vi "索引数据.vi"(5 "数据":T2[](array[typedef]), 6 "显示曲线范围":T3, 7 "显示数据":i32[](array[numeric]), 8 "测试类型":T1 caption="数据", 11 "索引簇":T4 {"索引" min=0}) -> (3 "数组":T5[](array[typedef]), 4 "当前索引":T2)   [LabVIEW 2020]
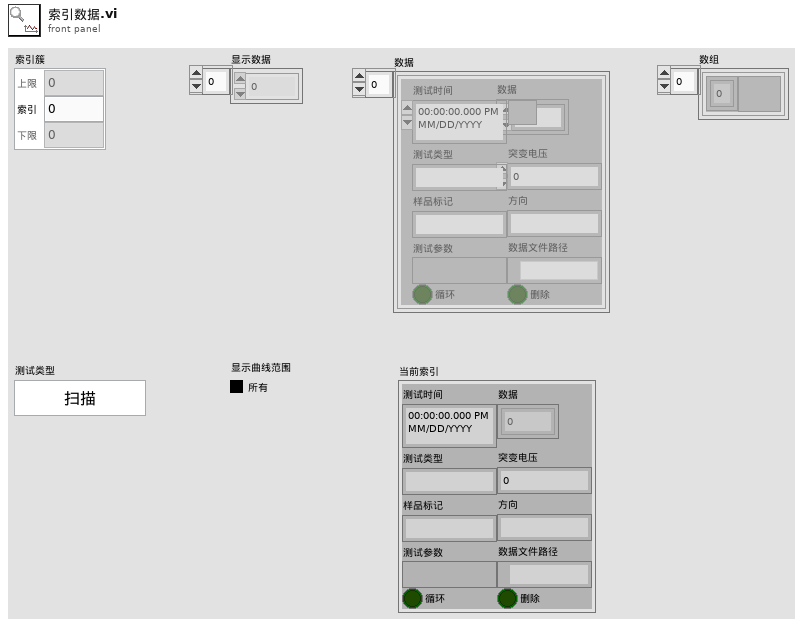
[diagram p1: front panel]
types:
  T1 = typedef "测试类型.ctl" = enum16{"扫描", "保持时间", "脉冲", "高速脉冲", "任意波形"}
  T2 = typedef "测试数据类型.ctl" = cluster{"测试时间":timestamp, "测试类型":string, "样品标记":string, "测试参数":variant, "循环":bool, "数据":dbl[][], "删除":bool, "突变电压":i32, "方向":string, "数据文件路径":path}
  T3 = typedef "显示曲线范围.ctl" = enum8{"False", "True", "Mixed"}
  T4 = typedef "索引簇.ctl" = cluster{"上限":i32, "索引":i32, "下限":i32}
  T5 = typedef "数据显示.xctl/波形数据定义.ctl" = cluster{"波形":dbl[][], "属性":variant}
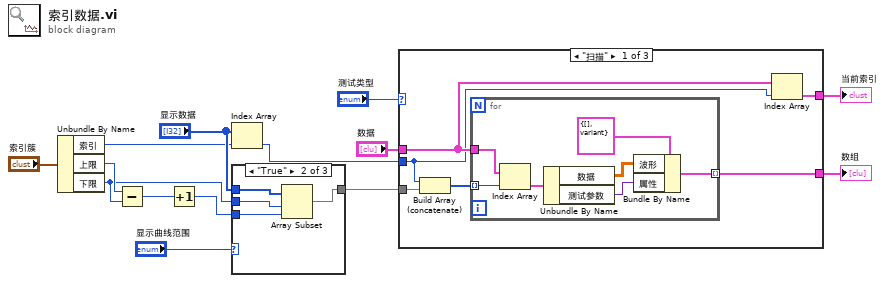
[diagram p0: block diagram]
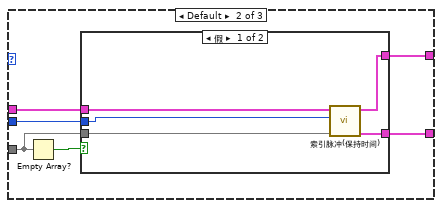
[diagram p2: hidden frame]
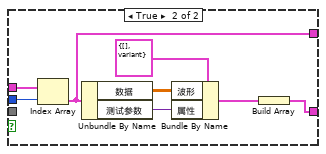
[diagram p3: hidden frame]
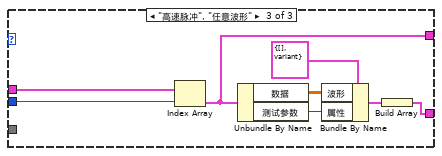
[diagram p4: hidden frame]
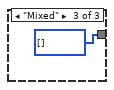
[diagram p6: hidden frame]
diagram:
  n1 = Unbundle By Name("索引簇") -> ("索引"=w6:i32, "上限"=w11:i32, "下限"=w10:i32)
  n2 = Subtract(x=w11, y=w10) -> (x-y=w9:i32)
  n3 = Increment(x=w9) -> (x+1=w1:i32)
  n4 = Index Array(array="显示数据", index=w6) -> (element=w4:i32)
  n5 = case shown="\"True\"" "显示曲线范围" {
    tunnel: "显示数据" -> [w15 w19 _]
    tunnel: w10 -> [_ w18 _]
    tunnel: w1 -> [_ w17 _]
    tunnel: [w15 w16 i32[] [] ("显示数据")] -> w8
    frame "False" {
    }
    frame "True" {
      n6 = Array Subset(array=w19, index=w18, length=w17) -> (w16:i32[])
    }
    frame "Mixed" {
    }
  }
  n7 = case shown="\"扫描\"" "测试类型" {
    tunnel: w8 -> [w26 w35 _]
    tunnel: [w25 w36 w54] -> w7
    tunnel: "数据" -> [w23 w39 w57]
    tunnel: w4 -> [w22 w38 w56]
    tunnel: [w21 w37 w53] -> w3
    frame "扫描" {
      n8 = Build Array (concatenate)(w22, w26) -> (w24:i32[])
      n9 = for {
        tunnel: w24 -> [w32] mode=indexing
        tunnel: w23 -> [w31]
        tunnel: [w27] -> w25 mode=indexing
        n10 = Index Array(array=w31, index=w32) -> (element=w33:T2)
        n11 = Unbundle By Name(w33) -> ("数据"=w30:dbl[][], "测试参数"=w29:variant)
        n12 = Bundle By Name(cluster=T5 {"波形"=[], "属性"=variant} ("波形数据"), "波形"=w30, "属性"=w29) -> (w27:T5)
      }
      n13 = Index Array(array=w23, index=w22) -> (element=w21:T2)
    }
    frame Default {
      n14 = Empty Array?(array=w35) -> (empty?=w34:bool)
      n15 = case shown="假" w34 {
        tunnel: w35 -> [w40 _]
        tunnel: w39 -> [w42 w48]
        tunnel: w38 -> [w41 w47]
        tunnel: [w44 w46] -> w37
        tunnel: [w43 w45] -> w36
        frame False {
          n16 = call "索引脉冲(保持时间).vi"("显示数据"=w40, "索引"=w41, "数据"=w42) -> ("数组"=w43:T5[], "测试数据"=w44:T2)  [unwired: 7 in]
        }
        frame True {
          n17 = Index Array(array=w48, index=w47) -> (element=w46:T2)
          n18 = Unbundle By Name(w46) -> ("数据"=w52:dbl[][], "测试参数"=w51:variant)
          n19 = Bundle By Name(cluster=T5 {"波形"=[], "属性"=variant} ("波形数据"), "波形"=w52, "属性"=w51) -> (w50:T5)
          n20 = Build Array(w50) -> (w45:T5[])
        }
      }
    }
    frame "高速脉冲", "任意波形" {
      n21 = Index Array(array=w57, index=w56) -> (element=w53:T2)
      n22 = Unbundle By Name(w53) -> ("数据"=w60:dbl[][], "测试参数"=w59:variant)
      n23 = Bundle By Name(cluster=T5 {"波形"=[], "属性"=variant} ("波形数据"), "波形"=w60, "属性"=w59) -> (w55:T5)
      n24 = Build Array(w55) -> (w54:T5[])
    }
  }
  "数组" <- w7
  "当前索引" <- w3
